vi "GUI_Lcave_AmplifierCams.vi"() -> ()   [LabVIEW 2013]
uses:
  shared programs/GUI_Template/GUI_master/tcp_new_data_event.ctl
  shared programs/GUI_Template/GUI_master/tcp new data cluster.ctl
  GUI_Stage_Cameras/Controls/Crosshair type def.ctl
  <userlib>/_OpenG.lib/array/array.llb/Filter 1D Array with Scalar (String)__ogtk.vi
panel:
  in  "Color Box":u32(colorbox)
  in  "TargetSize.Y::7":dbl=45.0 caption="y" min=2.0 max=3000.0 format="%#_6f"
  in  "TargetSize.X::7":dbl=47.0 caption="x" min=2.0 max=3000.0 format="%#_6f"
  in  "TargetSize.Y::6":dbl=45.0 caption="y" min=2.0 max=3000.0 format="%#_6f"
  in  "TargetSize.X::6":dbl=47.0 caption="x" min=2.0 max=3000.0 format="%#_6f"
  in  "TargetSize.Y::5":dbl=45.0 caption="y" min=2.0 max=3000.0 format="%#_6f"
  in  "TargetSize.X::5":dbl=47.0 caption="x" min=2.0 max=3000.0 format="%#_6f"
  in  "TargetSize.Y::4":dbl=45.0 caption="y" min=2.0 max=3000.0 format="%#_6f"
  in  "TargetSize.X::4":dbl=47.0 caption="x" min=2.0 max=3000.0 format="%#_6f"
  in  "TargetSize.Y::3":dbl=163.0 caption="y" min=2.0 max=3000.0 format="%#_6f"
  in  "TargetSize.X::3":dbl=152.0 caption="x" min=2.0 max=3000.0 format="%#_6f"
  in  "TargetSize.Y::2":dbl=74.0 caption="y" min=2.0 max=3000.0 format="%#_6f"
  in  "TargetSize.X::2":dbl=75.0 caption="x" min=2.0 max=3000.0 format="%#_6f"
  in  "active cams":string
  out "CCDs":string[](array[string])
  out "Cameras":T1
  in  "Target.Y::7":dbl=45.0 caption="y" min=0.0 max=2000.0 format="%#_6f"
  in  "Target.X::7":dbl=47.0 caption="x" min=0.0 max=2000.0 format="%#_6f"
  in  "Target.Y::6":dbl=45.0 caption="y" min=0.0 max=2000.0 format="%#_6f"
  in  "Target.X::6":dbl=47.0 caption="x" min=0.0 max=2000.0 format="%#_6f"
  in  "Target.Y::5":dbl=45.0 caption="y" min=0.0 max=2000.0 format="%#_6f"
  in  "Target.X::5":dbl=47.0 caption="x" min=0.0 max=2000.0 format="%#_6f"
  in  "Target.Y::4":dbl=45.0 caption="y" min=0.0 max=2000.0 format="%#_6f"
  in  "Target.X::4":dbl=47.0 caption="x" min=0.0 max=2000.0 format="%#_6f"
  in  "Target.Y::3":dbl=163.0 caption="y" min=0.0 max=2000.0 format="%#_6f"
  in  "Target.X::3":dbl=152.0 caption="x" min=0.0 max=2000.0 format="%#_6f"
  in  "Target.Y::2":dbl=74.0 caption="y" min=0.0 max=2000.0 format="%#_6f"
  in  "Target.X::2":dbl=75.0 caption="x" min=0.0 max=2000.0 format="%#_6f"
  out "error out":errorcluster
  out "image::7":T2(plugin-control) caption="GaiaImager2"
  in  "triggerdelay::7":dbl=0.001 caption="triggerdelay" min=0.0 max=0.09 format="%_4p"
  in  "triggerdelay::6":dbl=0.001 caption="triggerdelay" min=0.0 max=0.09 format="%_4p"
  in  "triggerdelay::5":dbl=0.001 caption="triggerdelay" min=0.0 max=0.09 format="%_4p"
  in  "triggerdelay::4":dbl=0.001 caption="triggerdelay" min=0.0 max=0.09 format="%_4p"
  in  "triggerdelay::3":dbl=0.001 caption="triggerdelay" min=0.0 max=0.09 format="%_4p"
  in  "triggerdelay::2":dbl=0.001 caption="triggerdelay" min=0.0 max=0.09 format="%_4p"
  in  "trigger::7":bool caption="Trigger"
  in  "centroidy::7":dbl=0.001 caption="centroid y" min=0.0 max=0.0 format="%_4f"
  in  "centroidx::7":dbl=0.001 caption="centroid x" min=0.0 max=0.0 format="%_4f"
  in  "exposure::7":dbl=0.001 caption="exposure" min=0.0001 max=1.0 format="%_4p"
  in  "GUIdevice 7":string="GaiaImager2"
  in  "trigger::6":bool caption="Trigger"
  in  "centroidy::6":dbl=0.001 caption="centroid y" min=0.0 max=0.0 format="%_4f"
  in  "centroidx::6":dbl=0.001 caption="centroid x" min=0.0 max=0.0 format="%_4f"
  in  "exposure::6":dbl=0.001 caption="exposure" min=0.0001 max=1.0 format="%_4p"
  out "image::6":T2(plugin-control) caption="BellaCam13_2"
  in  "GUIdevice 6":string="BellaCam13_2"
  in  "trigger::5":bool caption="Trigger"
  in  "centroidy::5":dbl=0.001 caption="centroid y" min=0.0 max=0.0 format="%_4f"
  in  "centroidx::5":dbl=0.001 caption="centroid x" min=0.0 max=0.0 format="%_4f"
  in  "exposure::5":dbl=0.001 caption="exposure" min=0.0001 max=1.0 format="%_4p"
  out "image::5":T2(plugin-control) caption="BellaCam16_3"
  in  "GUIdevice 5":string="BellaCam16_4"
  in  "trigger::4":bool caption="Trigger"
  in  "centroidy::4":dbl=0.001 caption="centroid y" min=0.0 max=0.0 format="%_4f"
  in  "centroidx::4":dbl=0.001 caption="centroid x" min=0.0 max=0.0 format="%_4f"
  in  "exposure::4":dbl=0.001 caption="exposure" min=0.0001 max=1.0 format="%_4p"
  out "image::4":T2(plugin-control) caption="BellaCam16_3"
  in  "GUIdevice 4":string="BellaCam16_3"
  in  "trigger::3":bool caption="Trigger"
  in  "centroidy::3":dbl=0.001 caption="centroid y" min=0.0 max=0.0 format="%_4f"
  in  "centroidx::3":dbl=0.001 caption="centroid x" min=0.0 max=0.0 format="%_4f"
  in  "exposure::3":dbl=0.001 caption="exposure" min=0.0001 max=1.0 format="%_4p"
  out "image::3":T2(plugin-control) caption="BellaCam16_2"
  in  "GUIdevice 3":string="BellaCam16_2"
  in  "trigger::2":bool caption="Trigger"
  in  "centroidy::2":dbl=0.001 caption="centroid y" min=0.0 max=0.0 format="%_4f"
  in  "centroidx::2":dbl=0.001 caption="centroid x" min=0.0 max=0.0 format="%_4f"
  in  "exposure::2":dbl=0.001 caption="exposure" min=0.0001 max=1.0 format="%_4p"
  out "image::2":T2(plugin-control) caption="BellaCam16_1"
  in  "GUIdevice 2":string="BellaCam16_1"
  out "tcp data event":T3
  in  "Refresh Button":bool caption="Update Crosshairs"
  in  "Select device":string(combo)="FrogHPD"
  in  "stop":bool
  in  "GUIdevice 1":string="HPD_CCD"
  # "XHair location"
  # "XHair size"
  # "XHair location"
  # "XHair size"
  # "XHair location"
  # "XHair size"
  # "XHair location"
  # "XHair size"
  # "XHair location"
  # "XHair size"
  # "XHair location"
  # "XHair size"
  # "XHair location"
  # "XHair size"
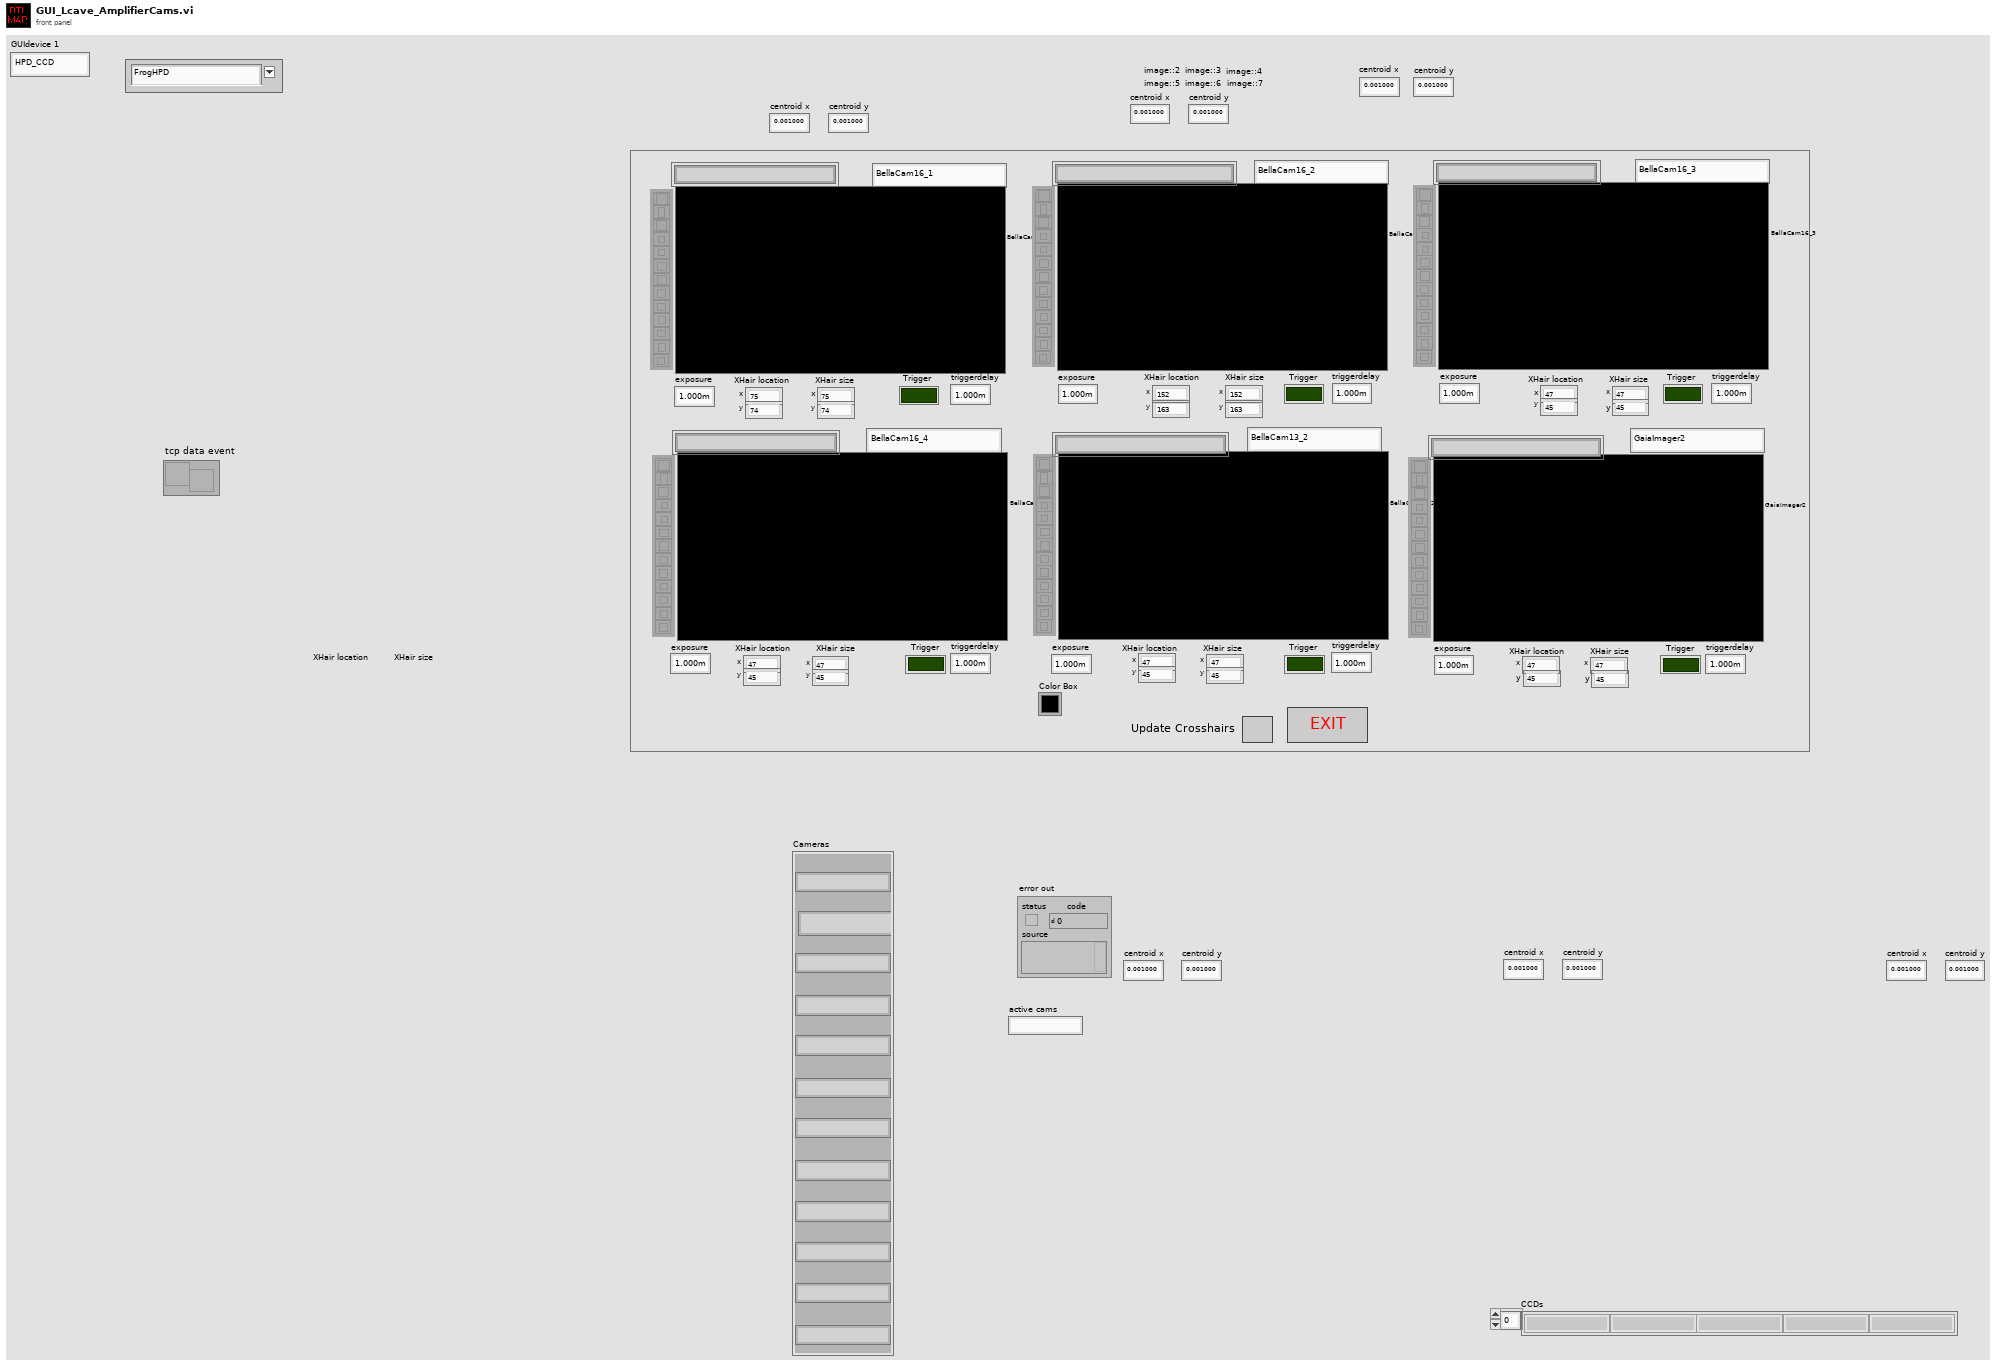
[diagram p1: front panel]
types:
  T1 = cluster{"[0]":string, "[1]":string, "[2]":string, "[3]":string, "[4]":string, "[5]":string, "[6]":string, "[7]":string, "[8]":string, "[8] 2":string, "[8] 3":string, "[8] 4":string}
  T2 = typedef "IMAQ Image.ctl" = refnum<image>
  T3 = typedef "tcp_new_data_event.ctl" = refnum<user-event>
  T4 = typedef "Image Type" = u32
  T5 = cluster{"TargetSize.X::2":refnum<vi>, "TargetSize.Y::2":refnum<vi>}
  T6 = cluster{"TargetSize.X::3":refnum<vi>, "TargetSize.Y::3":refnum<vi>}
  T7 = cluster{"TargetSize.X::4":refnum<vi>, "TargetSize.Y::4":refnum<vi>}
  T8 = cluster{"TargetSize.X::5":refnum<vi>, "TargetSize.Y::5":refnum<vi>}
  T9 = cluster{"TargetSize.X::6":refnum<vi>, "TargetSize.Y::6":refnum<vi>}
  T10 = cluster{"TargetSize.X::7":refnum<vi>, "TargetSize.Y::7":refnum<vi>}
  T11 = cluster{"Target.X::2":refnum<vi>, "Target.Y::2":refnum<vi>}
  T12 = cluster{"Target.X::3":refnum<vi>, "Target.Y::3":refnum<vi>}
  T13 = cluster{"Target.X::4":refnum<vi>, "Target.Y::4":refnum<vi>}
  T14 = cluster{"Target.X::5":refnum<vi>, "Target.Y::5":refnum<vi>}
  T15 = cluster{"Target.X::6":refnum<vi>, "Target.Y::6":refnum<vi>}
  T16 = cluster{"Target.X::7":refnum<vi>, "Target.Y::7":refnum<vi>}
  T17 = cluster{"[0]":string, "[1]":string, "[2]":string, "[3]":string, "[4]":string, "[5]":string, "[6]":string, "[7]":string, "[8]":string, "[9]":string, "[10]":string, "[11]":string}
  T18 = cluster{"TargetSize.X::7":refnum<vi>, "TargetSize.Y::7":refnum<vi>}[]
  T19 = cluster{"Target.X::7":refnum<vi>, "Target.Y::7":refnum<vi>}[]
  T20 = typedef "Crosshair type def.ctl" = cluster{"Draw":bool, "Target":cluster{"x":dbl, "y":dbl}, "Size":cluster{"x":dbl, "y":dbl}, "Angle":dbl, "Color":u32}
  T21 = cluster{"Left":i32, "Top":i32, "Right":i32, "Bottom":i32}
  T22 = enum32{"invalid app kind", "Development System", "Run Time System", "Student Edition", "Embedded LabVIEW", "Evaluation", "Custom"}
  T23 = typedef "tcp new data cluster.ctl" = cluster{"EventEnum":enum16{"new data", "connection status update"}, "Device name":string}
  T24 = enum32{"Invalid", "Standard", "Closed", "Hidden", "Minimized", "Maximized"}
  T25 = cluster{"Core":cluster{"Current VI Reference":refnum<vi>, "Close Panel on Exit?":bool}, "Your Boolean data":bool, "active cams":string, "SuperGUI":cluster{"STOP queue":refnum<queue>, "SuperGUI ref":refnum<vi>}}
  T26 = cluster{"STOP queue":refnum<queue>, "SuperGUI ref":refnum<vi>}
  T27 = cluster{"Current VI Reference":refnum<vi>, "Close Panel on Exit?":bool}
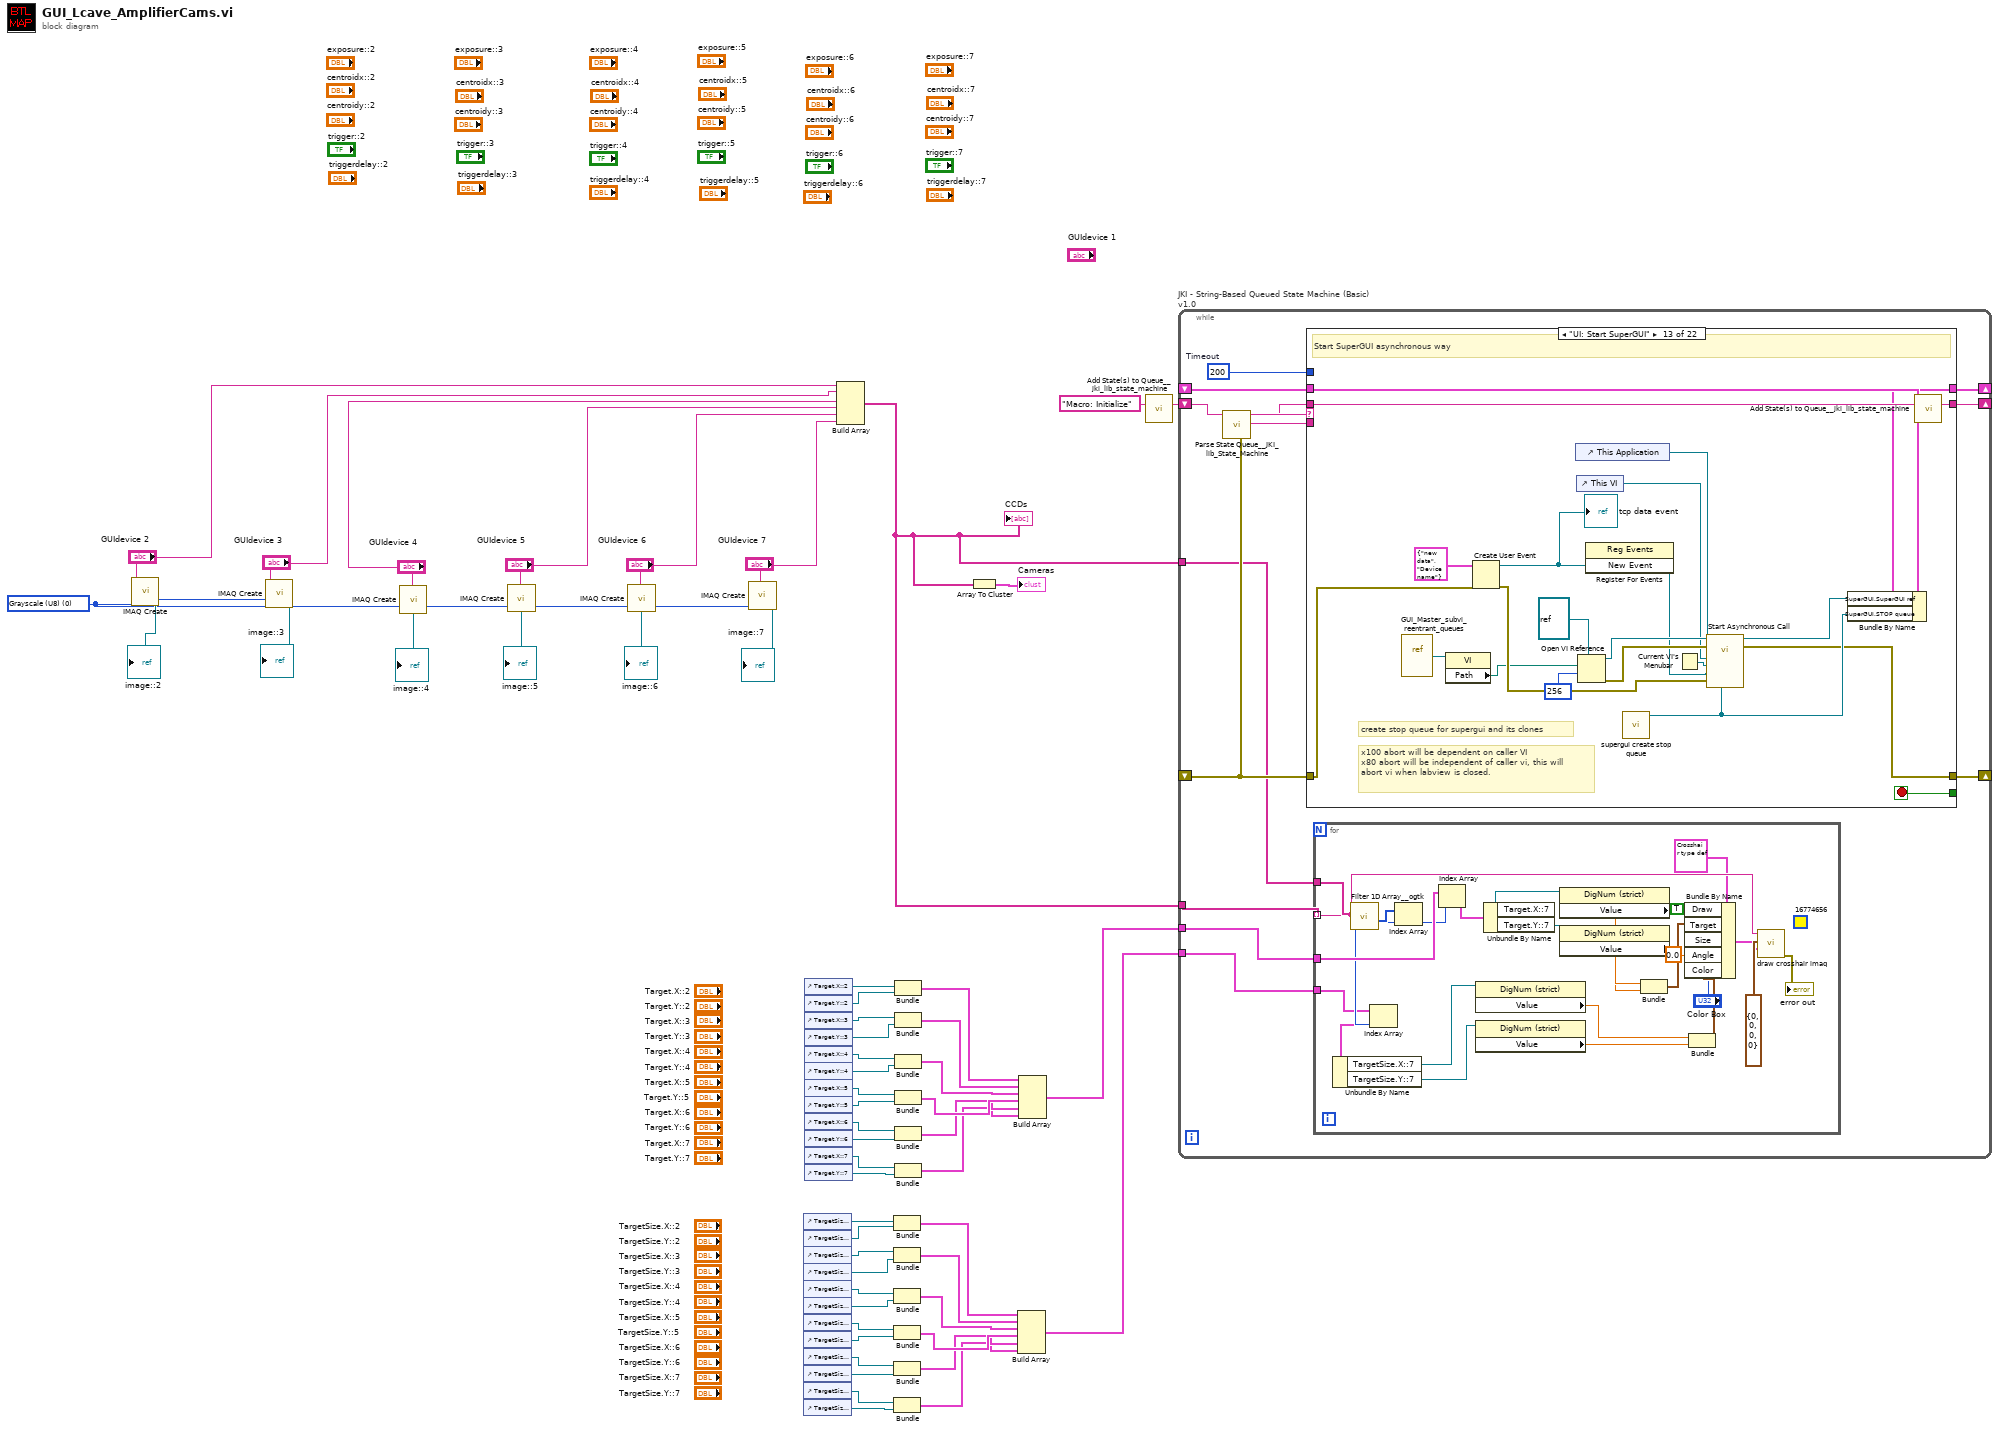
[diagram p0: block diagram]
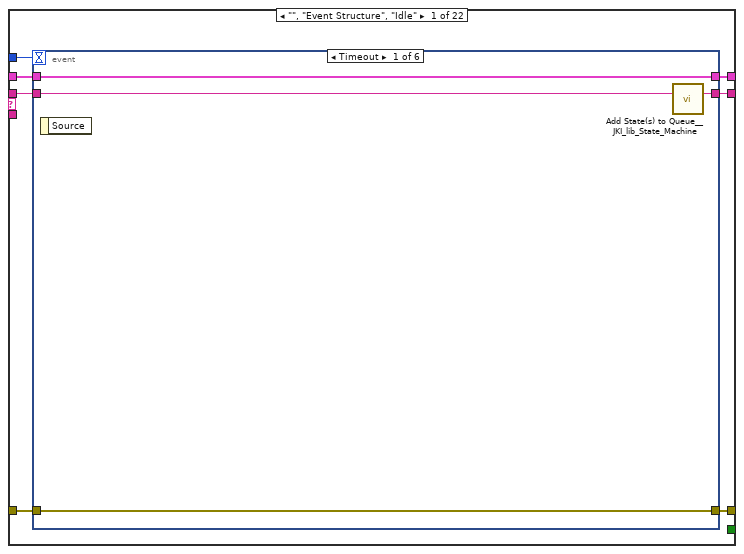
[diagram p2: hidden frame]
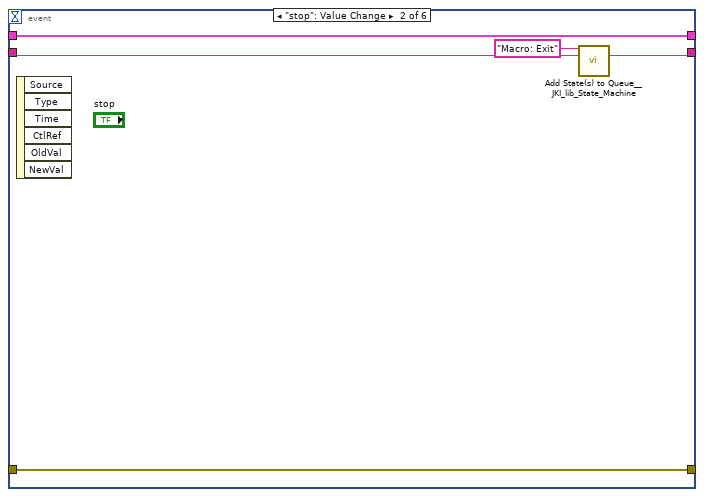
[diagram p3: hidden frame]
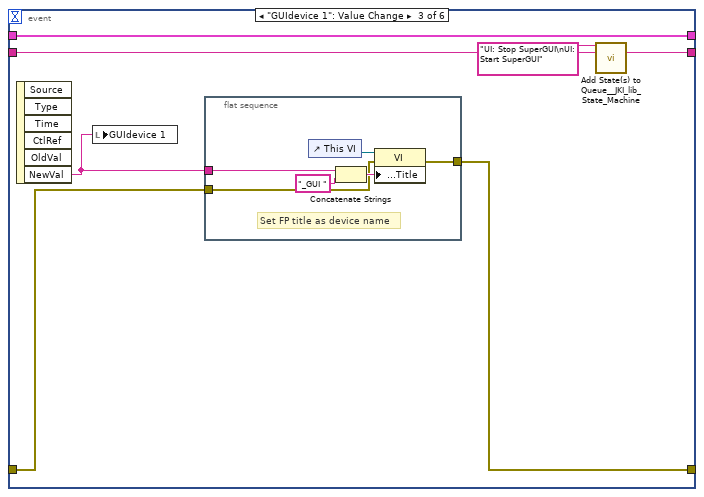
[diagram p4: hidden frame]
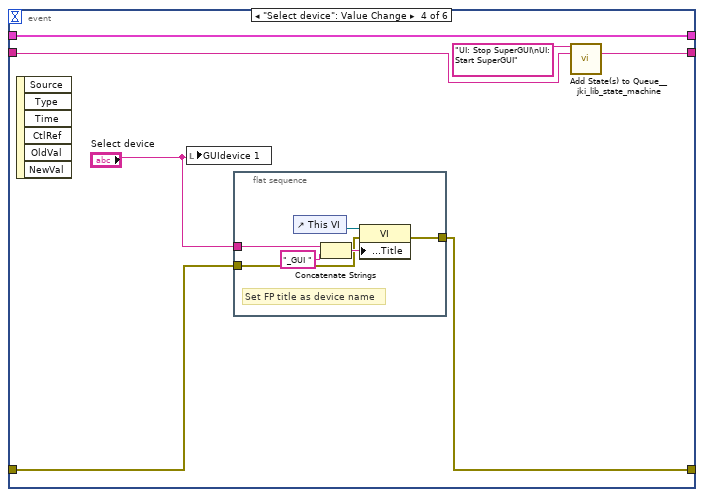
[diagram p5: hidden frame]
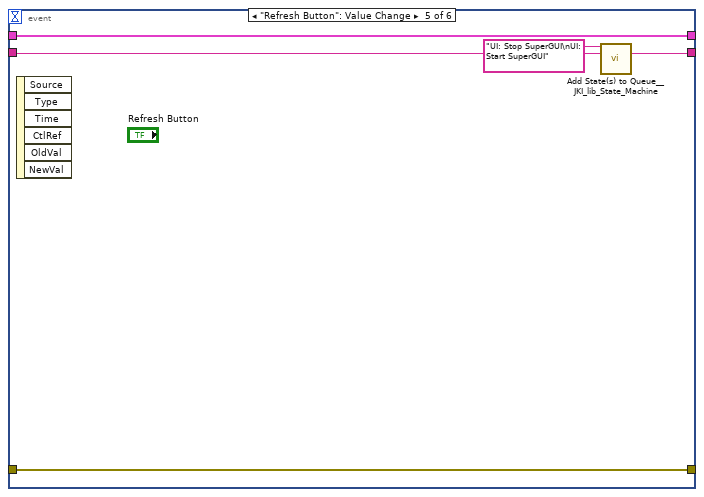
[diagram p6: hidden frame]
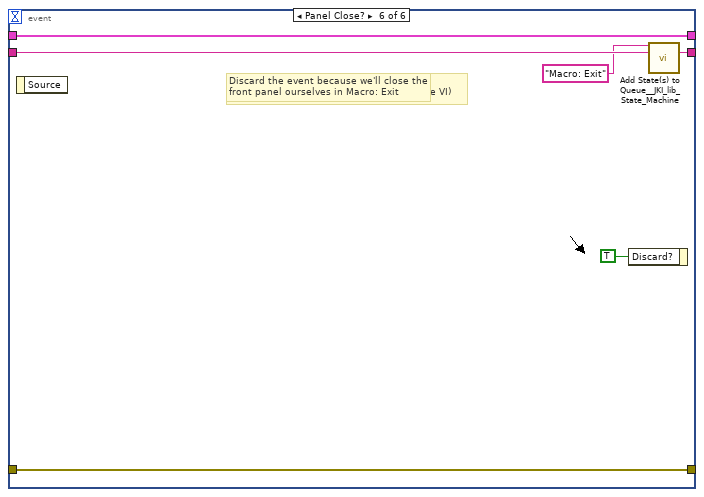
[diagram p7: hidden frame]
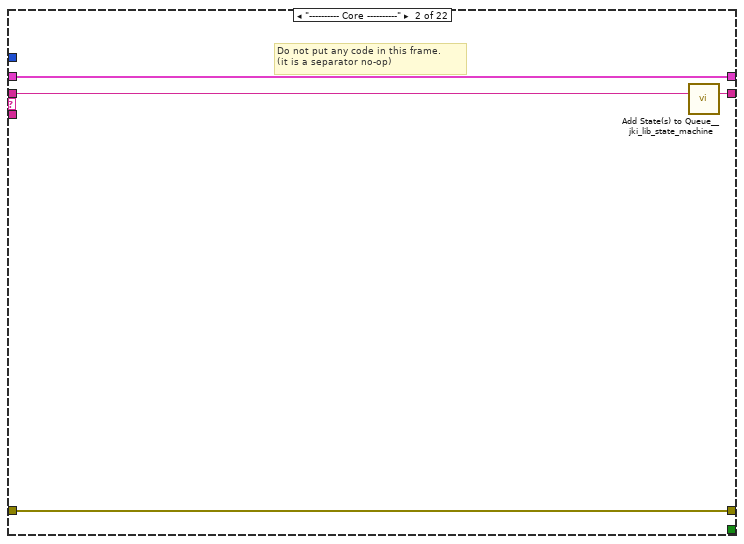
[diagram p8: hidden frame]
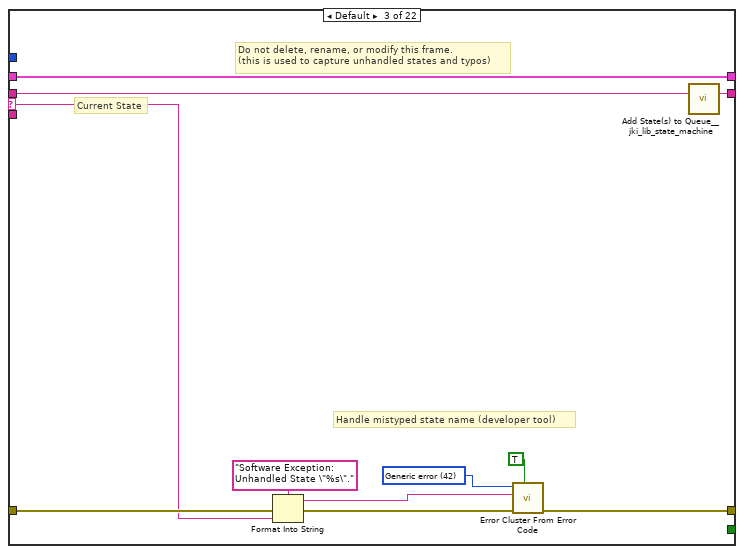
[diagram p9: hidden frame]
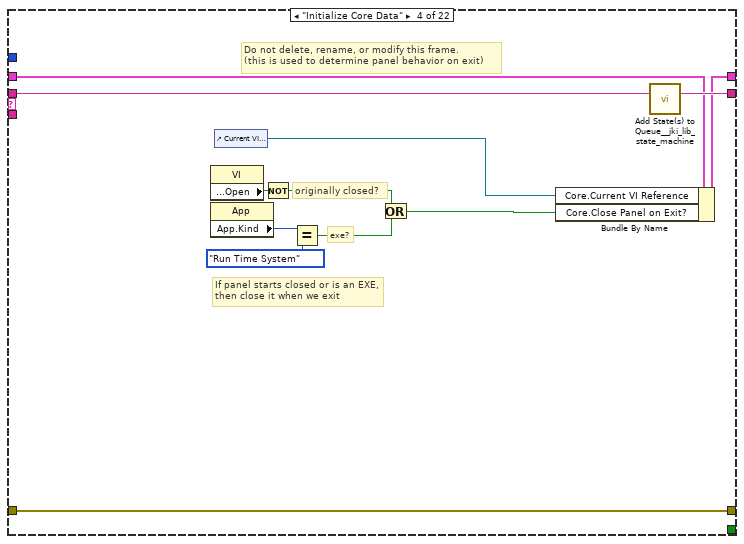
[diagram p10: hidden frame]
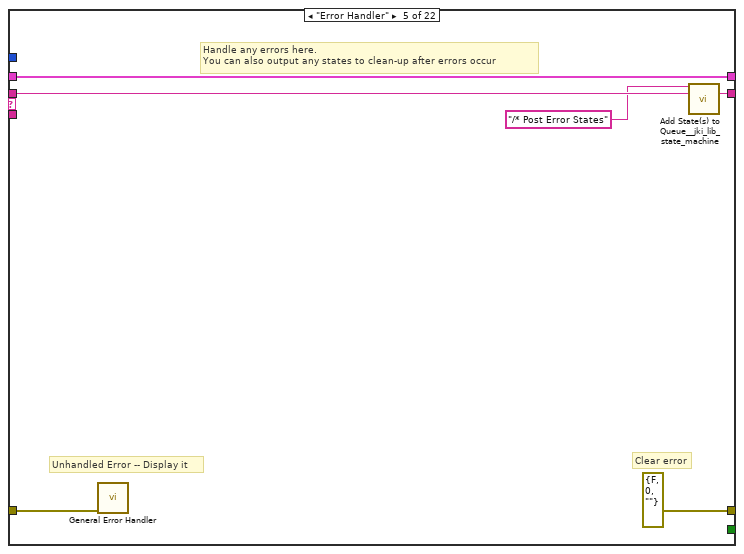
[diagram p11: hidden frame]
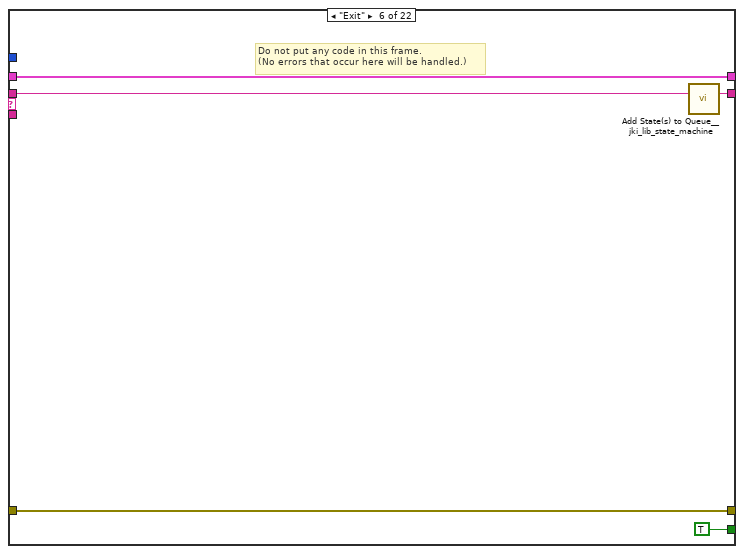
[diagram p12: hidden frame]
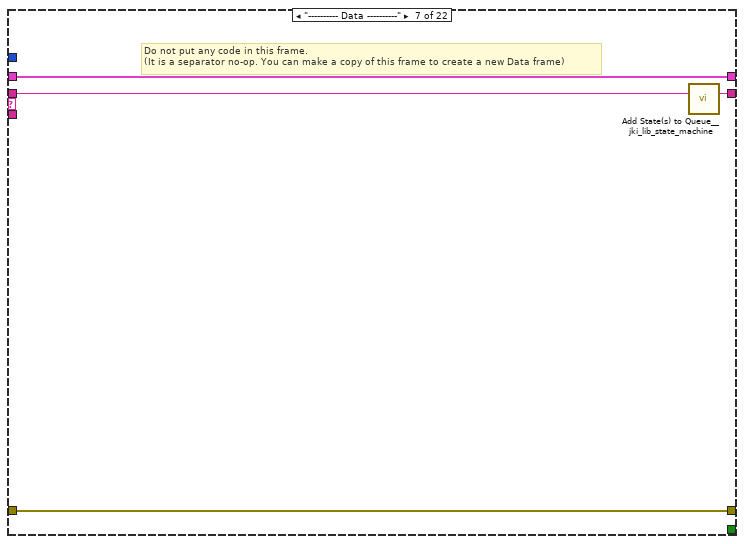
[diagram p13: hidden frame]
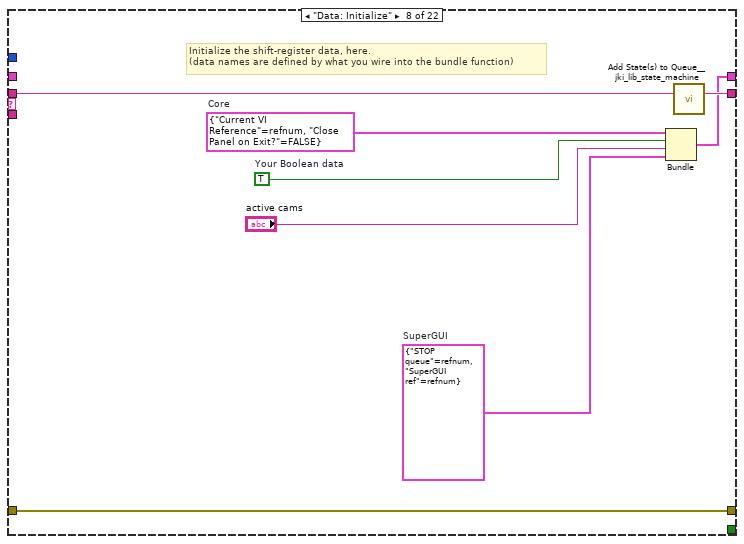
[diagram p14: hidden frame]
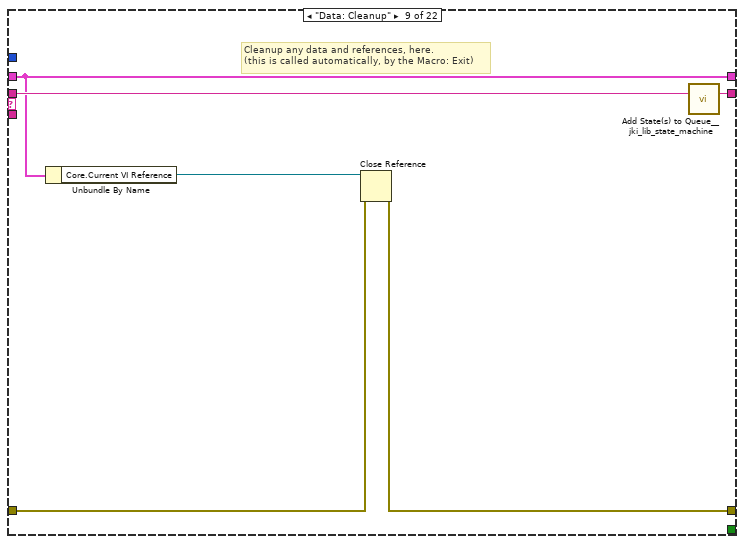
[diagram p15: hidden frame]
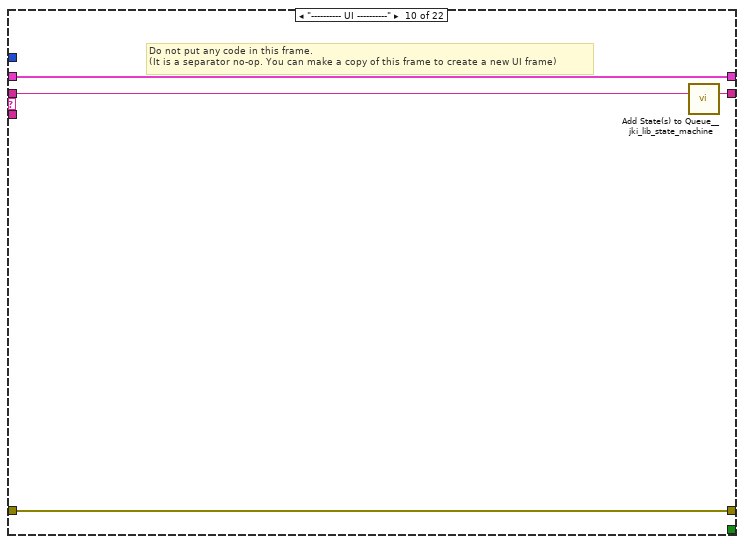
[diagram p16: hidden frame]
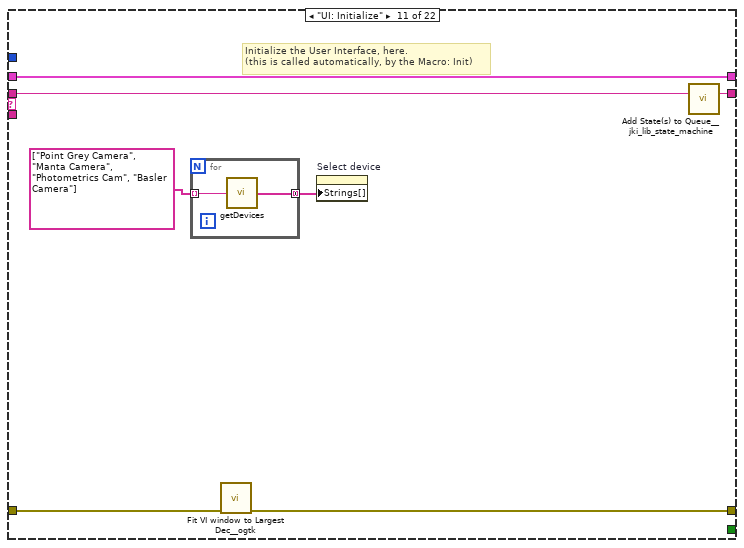
[diagram p17: hidden frame]
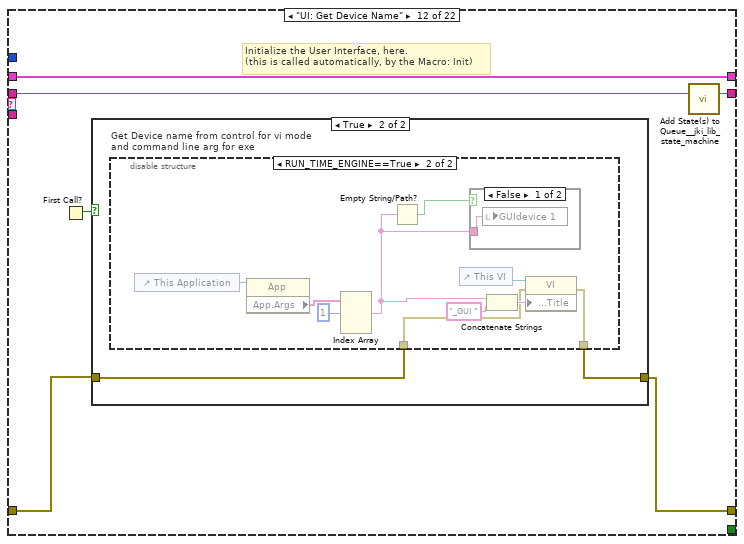
[diagram p18: hidden frame]
diagram:
  w48 = T4 0 items=["Grayscale (U8)", "Grayscale (I16)", "Grayscale (SGL)", "Complex (CSG)", "RGB (U32)", "HSL (U32)", "RGB (U64)", "Grayscale (U16)"] ("Image Type")
  n1 = call "IMAQ Create"("Image Name"="GUIdevice 2", "Image Type"=w48) -> ("New Image"=→"image::2":T2)  [unwired: 3 in, 1 out]
  n2 = call "IMAQ Create"("Image Name"="GUIdevice 3", "Image Type"=w48) -> ("New Image"=→"image::3":T2)  [unwired: 3 in, 1 out]
  n3 = call "IMAQ Create"("Image Name"="GUIdevice 4", "Image Type"=w48) -> ("New Image"=→"image::4":T2)  [unwired: 3 in, 1 out]
  n4 = call "IMAQ Create"("Image Name"="GUIdevice 5", "Image Type"=w48) -> ("New Image"=→"image::5":T2)  [unwired: 3 in, 1 out]
  n5 = call "IMAQ Create"("Image Name"="GUIdevice 6", "Image Type"=w48) -> ("New Image"=→"image::6":T2)  [unwired: 3 in, 1 out]
  n6 = call "IMAQ Create"("Image Name"="GUIdevice 7", "Image Type"=w48) -> ("New Image"=→"image::7":T2)  [unwired: 3 in, 1 out]
  n7 = control-ref of="TargetSize.X::2"() -> (w19:refnum<vi>)
  n8 = control-ref of="TargetSize.Y::2"() -> (w18:refnum<vi>)
  n9 = control-ref of="TargetSize.X::3"() -> (w17:refnum<vi>)
  n10 = control-ref of="TargetSize.Y::3"() -> (w16:refnum<vi>)
  n11 = control-ref of="TargetSize.X::4"() -> (w15:refnum<vi>)
  n12 = control-ref of="TargetSize.Y::4"() -> (w14:refnum<vi>)
  n13 = control-ref of="TargetSize.X::5"() -> (w13:refnum<vi>)
  n14 = control-ref of="TargetSize.Y::5"() -> (w12:refnum<vi>)
  n15 = control-ref of="TargetSize.X::6"() -> (w11:refnum<vi>)
  n16 = control-ref of="TargetSize.Y::6"() -> (w10:refnum<vi>)
  n17 = control-ref of="TargetSize.X::7"() -> (w9:refnum<vi>)
  n18 = control-ref of="TargetSize.Y::7"() -> (w8:refnum<vi>)
  n19 = control-ref of="Target.X::2"() -> (w46:refnum<vi>)
  n20 = control-ref of="Target.Y::2"() -> (w45:refnum<vi>)
  n21 = control-ref of="Target.X::3"() -> (w44:refnum<vi>)
  n22 = control-ref of="Target.Y::3"() -> (w43:refnum<vi>)
  n23 = control-ref of="Target.X::4"() -> (w42:refnum<vi>)
  n24 = control-ref of="Target.Y::4"() -> (w41:refnum<vi>)
  n25 = control-ref of="Target.X::5"() -> (w40:refnum<vi>)
  n26 = control-ref of="Target.Y::5"() -> (w39:refnum<vi>)
  n27 = control-ref of="Target.X::6"() -> (w38:refnum<vi>)
  n28 = control-ref of="Target.Y::6"() -> (w37:refnum<vi>)
  n29 = control-ref of="Target.X::7"() -> (w36:refnum<vi>)
  n30 = control-ref of="Target.Y::7"() -> (w35:refnum<vi>)
  n31 = Build Array("GUIdevice 2", "GUIdevice 3", "GUIdevice 4", "GUIdevice 5", "GUIdevice 6", "GUIdevice 7") -> (w20:string[])
  "CCDs" <- w20
  n32 = Bundle("TargetSize.X::2"=w19, "TargetSize.Y::2"=w18) -> (w7:T5)  [unwired: 1 in]
  n33 = Bundle("TargetSize.X::3"=w17, "TargetSize.Y::3"=w16) -> (w6:T6)  [unwired: 1 in]
  n34 = Bundle("TargetSize.X::4"=w15, "TargetSize.Y::4"=w14) -> (w2:T7)  [unwired: 1 in]
  n35 = Bundle("TargetSize.X::5"=w13, "TargetSize.Y::5"=w12) -> (w5:T8)  [unwired: 1 in]
  n36 = Bundle("TargetSize.X::6"=w11, "TargetSize.Y::6"=w10) -> (w4:T9)  [unwired: 1 in]
  n37 = Bundle("TargetSize.X::7"=w9, "TargetSize.Y::7"=w8) -> (w3:T10)  [unwired: 1 in]
  n38 = Bundle("Target.X::2"=w46, "Target.Y::2"=w45) -> (w34:T11)  [unwired: 1 in]
  n39 = Bundle("Target.X::3"=w44, "Target.Y::3"=w43) -> (w33:T12)  [unwired: 1 in]
  n40 = Bundle("Target.X::4"=w42, "Target.Y::4"=w41) -> (w29:T13)  [unwired: 1 in]
  n41 = Bundle("Target.X::5"=w40, "Target.Y::5"=w39) -> (w32:T14)  [unwired: 1 in]
  n42 = Bundle("Target.X::6"=w38, "Target.Y::6"=w37) -> (w31:T15)  [unwired: 1 in]
  n43 = Bundle("Target.X::7"=w36, "Target.Y::7"=w35) -> (w30:T16)  [unwired: 1 in]
  n44 = Array To Cluster(array=w20) -> (cluster=→"Cameras":T17)
  n45 = Build Array(w7, w6, w2, w5, w4, w3) -> (w1:T18)
  n46 = Build Array(w34, w33, w29, w32, w31, w30) -> (w28:T19)
  n47 = call <vilib>:"Add State(s) to Queue__jki_lib_state_machine.vi"("State(s) in (\"\")"="Macro: Initialize") -> ("States Out"=w55:string)  [unwired: 14 in]
  n48 = while "JKI - String-Based Queued State Machine (Basic) v1.0" {
    shift-right: [w63] -> _
    shift-left: _ -> [w58]
    shift-right: [w66] -> _
    shift-left: _ -> [w61]
    shift-right: [w65] -> _
    shift-left: w55 -> [w67]
    tunnel: w28 -> [w60]
    tunnel: w20 -> [w59]
    tunnel: w20 -> [w57]
    tunnel: w1 -> [w56]
    stop <- w64 stop-if-true
    w62 = 200  # Timeout
    n49 = call <vilib>:"Parse State Queue__JKI_lib_State_Machine.vi"("State Queue"=w67, "Error In (no error)"=w61) -> ("Remaining States"=w69:string, "Current State"=w70:string, "Arguments"=w68:string)  [unwired: 11 in]
    n50 = case shown="\"UI: Start SuperGUI\"" w70 {
      selector: w70 -> [_ _ w153 _ _ _ _ _ _ _ _ _ _ _ _ _ _ _ _ _ _ _]
      tunnel: w69 -> [w102 w152 w157 w175 w181 w186 w190 w198 w204 w208 w215 w223 w258 w266 w272 w283 w309 w314 w324 w328 w332 w336]
      tunnel: w68 -> [_ _ _ _ _ _ _ _ _ _ _ _ _ _ w267 w277 _ _ _ _ _ _]
      tunnel: w58 -> [w100 w149 w155 w166 w178 w184 w187 _ w199 w205 w213 w221 w249 w261 w270 w279 w306 w311 w321 w325 w329 w333]
      tunnel: [w99 w150 w159 w172 errorcluster {"status"=FALSE, "code"=0, "source"=""} ("error out") w183 w188 w195 w200 w206 w211 w218 w242 w259 w268 w280 w307 w312 w322 w326 w330 w334] -> w66
      tunnel: w61 -> [w98 w150 w158 w172 w177 w183 w188 w195 w201 w206 w212 w219 w243 w260 w269 w281 w307 w312 w322 w326 w330 w334]
      tunnel: [w101 w151 w156 w174 w180 w185 w189 w197 w203 w207 w214 w222 w257 w265 w271 w282 w308 w313 w323 w327 w331 w335] -> w65
      tunnel: [_ _ _ _ _ TRUE _ _ _ _ _ _ _ _ _ _ _ _ _ _ _ _] -> w64
      tunnel: [w97 w149 w155 w173 w178 w184 w187 w196 w199 w205 w213 w221 w248 w261 w270 w279 w306 w311 w321 w325 w329 w333] -> w63
      tunnel: w62 -> [w96 _ _ _ _ _ _ _ _ _ _ _ _ _ _ _ _ _ _ _ _ _]
      frame "", "Event Structure", "Idle" {
        n51 = event shown="[0] Timeout" {
          selector: _ -> [_ _ _ _ _ _]
          dyn-events: _ -> [_ _ _ _ _ _]
          timeout: w96 -> [_ _ _ _ _ _]
          tunnel: w102 -> [w106 w109 w115 w127 w140 w148]
          tunnel: [w105 w108 w114 w126 w139 w147] -> w101
          tunnel: w100 -> [w103 w111 w118 w131 w142 w145]
          tunnel: [w104 w110 w116 w129 w141 w146] -> w99
          tunnel: w98 -> [w104 w110 w117 w130 w141 w146]
          tunnel: [w103 w111 w118 w131 w142 w145] -> w97
          event Timeout {
            n52 = event-data() -> ()  [unwired: 1 in, 1 out]
            n53 = call <vilib>:"Add State(s) to Queue__JKI_lib_State_Machine.vi"("State(s) in (\"\")"=w106) -> ("States Out"=w105:string)  [unwired: 14 in]
          }
          event "stop": Value Change {
            n54 = event-data() -> ()  [unwired: 1 in, 6 out]
            n55 = call <vilib>:"Add State(s) to Queue__JKI_lib_State_Machine.vi"("State(s) in Front (\"\")"="Macro: Exit", "State(s) in (\"\")"=w109) -> ("States Out"=w108:string)  [unwired: 13 in]
          }
          event "GUIdevice 1": Value Change {
            n56 = event-data() -> ("NewVal"=w112:string)  [unwired: 1 in, 5 out]
            n57 = local write "GUIdevice 1"(w112) -> ()
            n58 = flat-sequence {
              tunnel: [w121] -> w116
              tunnel: w117 -> [w120]
              tunnel: w112 -> [w119]
              frame #0 {
                # "Set FP title as device name"
                n59 = control-ref of="This VI"() -> (w124:refnum<vi>)
                n60 = Concatenate Strings(w119, "_GUI ") -> (w123:string)
                n61 = property class="VI"(reference=w124, error in=w120, "Front Panel.Title"=w123) -> (error out=w121:errorcluster)  [unwired: 1 out]
              }
            }
            n62 = call <vilib>:"Add State(s) to Queue__JKI_lib_State_Machine.vi"("State(s) in Front (\"\")"="UI: Stop SuperGUI\nUI: Start SuperGUI", "State(s) in (\"\")"=w115) -> ("States Out"=w114:string)  [unwired: 13 in]
          }
          event "Select device": Value Change {
            n63 = event-data() -> ()  [unwired: 1 in, 6 out]
            n64 = local write "GUIdevice 1"("Select device") -> ()
            n65 = flat-sequence {
              tunnel: [w134] -> w129
              tunnel: w130 -> [w133]
              tunnel: "Select device" -> [w132]
              frame #0 {
                # "Set FP title as device name"
                n66 = control-ref of="This VI"() -> (w137:refnum<vi>)
                n67 = Concatenate Strings(w132, "_GUI ") -> (w136:string)
                n68 = property class="VI"(reference=w137, error in=w133, "Front Panel.Title"=w136) -> (error out=w134:errorcluster)  [unwired: 1 out]
              }
            }
            n69 = call <vilib>:"Add State(s) to Queue__jki_lib_state_machine.vi"("State(s) in Front (\"\")"="UI: Stop SuperGUI\nUI: Start SuperGUI", "State(s) in (\"\")"=w127) -> ("States Out"=w126:string)  [unwired: 13 in]
          }
          event "Refresh Button": Value Change {
            n70 = event-data() -> ()  [unwired: 1 in, 6 out]
            n71 = call <vilib>:"Add State(s) to Queue__JKI_lib_State_Machine.vi"("State(s) in Front (\"\")"="UI: Stop SuperGUI\nUI: Start SuperGUI", "State(s) in (\"\")"=w140) -> ("States Out"=w139:string)  [unwired: 13 in]
          }
          event Panel Close? {
            # "Discard the event because we'll close the front panel ourselves in Macro: Exit"
            # "Close Panel button (pressed) Event\n(this executes Macro: Exit to terminate the VI)"
            n72 = event-data() -> ()  [unwired: 1 in, 1 out]
            n73 = event-data("Discard?"=TRUE) -> ()  [unwired: 1 in, 1 out]
            n74 = call <vilib>:"Add State(s) to Queue__JKI_lib_State_Machine.vi"("State(s) in Front (\"\")"="Macro: Exit", "State(s) in (\"\")"=w148) -> ("States Out"=w147:string)  [unwired: 13 in]
          }
        }
      }
      frame "---------- Core ----------" {
        # "Do not put any code in this frame.\n(it is a separator no-op)"
        n75 = call <vilib>:"Add State(s) to Queue__jki_lib_state_machine.vi"("State(s) in (\"\")"=w152) -> ("States Out"=w151:string)  [unwired: 14 in]
      }
      frame Default {
        w162 = 42 items=["No error", "Argument error", "Memory is full", "Out of zone", "End of file", "File already open", "Generic file I/O error", "File not found", "File permission error", "Disk is full", "Duplicate path", "Too many files open", "System feature not enabled", "Resource file not found", "Cannot add resource", "Resource not found", "Image not found", "Image memory error", "Pen does not exist", "Config type invalid", "Config token not found", "Config parse error", "Config memory error", "Bad external code format", "Bad external code offset", "External code not present", "Null window", "Destroy window error", "Null menu", "Print aborted", "Bad print record", "Print driver error", "Windows error during printing", "Memory error during printing", "Print dialog error", "Generic print error", "Invalid device refnum", "Device not found", "Device parameter error", "Device unit error", "Cannot open device", "Device call aborted", "Generic error", "Cancelled by user", "Object ID too low", "Object ID too high", "Object not in heap", "Unknown heap", "Unknown object (invalid DefProc)", "Unknown object (DefProc not in table)", "Message out of range", "Invalid (null) method", "Unknown message", "Manager call not supported", "Bad address", "Network operation in progress", "Network operation timed out", "Connection is busy", "Network attribute not supported", "Network error", "Address in use", "System out of memory", "Connection aborted", "Connection refused", "Not connected", "Already connected", "Connection closed", "Initialization error (interapplication manager)", "Bad occurrence", "Wait on unbound occurrence handler", "Occurrence queue overflow", "Datalog type conflict", "Unused", "Unrecognized type (interapplication manager)", "Memory corrupt", "Failed to make temporary DLL", "Old CIN version", "Drag socket not found", "Failed to load drop-object", "Failed to register OLE object", "Failed to release OLE object", "Format specifier type mismatch", "Unknown format specifier", "Too few format specifiers", "Too many format specifiers", "Scan failed", "Newer CIN version", "Error converting to variant", "Runtime menu error", "Password tampered", "Variant attribute not found", "Incompatible variant data type", "Event data is not available", "Event Store is not present", "Occurrence is not found", "Event Queue is not created", "Event info is not available", "Refnum passed is NULL", "Error retrieving Class GUID", "Error retrieving CoClass GUID", "Error retrieving TypeLib GUID.", "Bad built application magic bytes.", "Specific driver is different from the specific driver associated with the Logical Name.", "There is no session opened to the class driver.", "Max Error", "MAX - Error with config objects", "MAX - Error loading configuration", "MAX - Group not supported"]
        # "Current State"
        # "Do not delete, rename, or modify this frame.\n(this is used to capture unhandled states and typos)"
        # "Handle mistyped state name (developer tool)"
        n76 = Format Into String(format string="Software Exception: Unhandled State \"%s\"." ("message"), error in=w158, w153) -> (resulting string=w161:string, error out=w160:errorcluster)  [unwired: 1 in]
        n77 = call <vilib>:"Error Cluster From Error Code.vi"("show call chain? (False)"=TRUE, "error in (no error)"=w160, "error message (\"\")"=w161, "error code (0)"=w162) -> ("error out"=w159:errorcluster)  [unwired: 5 in]
        n78 = call <vilib>:"Add State(s) to Queue__jki_lib_state_machine.vi"("State(s) in (\"\")"=w157) -> ("States Out"=w156:string)  [unwired: 14 in]
      }
      frame "Initialize Core Data" {
        # "Do not delete, rename, or modify this frame.\n(this is used to determine panel behavior on exit)"
        # "originally closed?"
        # "exe?"
        # "If panel starts closed or is an EXE, then close it when we exit"
        n79 = property class="VI"() -> ("Front Panel.Open"=w171:bool)  [unwired: 2 in, 2 out]
        n80 = property class="App"() -> ("App.Kind"=w170:T22)  [unwired: 2 in, 2 out]
        n81 = control-ref of="Current VI Reference"() -> (w164:refnum<vi>)
        n82 = Not(x=w171) -> (.not. x?=w168:bool)
        n83 = Equal?(x=w170, y=T22."Run Time System" ("Application:Kind")) -> (x = y?=w167:bool)
        n84 = Or(x=w168, y=w167) -> (x .or. y?=w165:bool)
        n85 = Bundle By Name(cluster=w166, "Core.Current VI Reference"=w164, "Core.Close Panel on Exit?"=w165) -> (w173:T25)
        n86 = call <vilib>:"Add State(s) to Queue__jki_lib_state_machine.vi"("State(s) in (\"\")"=w175) -> ("States Out"=w174:string)  [unwired: 14 in]
      }
      frame "Error Handler" {
        # "Unhandled Error -- Display it"
        # "Handle any errors here.\nYou can also output any states to clean-up after errors occur"
        # "Clear error"
        n87 = call <vilib>:"General Error Handler.vi"("error in (no error)"=w177) -> ()  [unwired: 10 in, 5 out]
        n88 = call <vilib>:"Add State(s) to Queue__jki_lib_state_machine.vi"("State(s) in Front (\"\")"="/* Post Error States", "State(s) in (\"\")"=w181) -> ("States Out"=w180:string)  [unwired: 13 in]
      }
      frame "Exit" {
        # "Do not put any code in this frame.\n(No errors that occur here will be handled.)"
        n89 = call <vilib>:"Add State(s) to Queue__jki_lib_state_machine.vi"("State(s) in (\"\")"=w186) -> ("States Out"=w185:string)  [unwired: 14 in]
      }
      frame "---------- Data ----------" {
        # "Do not put any code in this frame.\n(It is a separator no-op. You can make a copy of this frame to create a new Data frame)"
        n90 = call <vilib>:"Add State(s) to Queue__jki_lib_state_machine.vi"("State(s) in (\"\")"=w190) -> ("States Out"=w189:string)  [unwired: 14 in]
      }
      frame "Data: Initialize" {
        w191 = T26 {"STOP queue"=refnum, "SuperGUI ref"=refnum}  # SuperGUI
        w192 = T27 {"Current VI Reference"=refnum, "Close Panel on Exit?"=FALSE}  # Core
        w194 = TRUE  # Your Boolean data
        # "Initialize the shift-register data, here.\n(data names are defined by what you wire into the bundle function)"
        n91 = Bundle("Core"=w192, "Your Boolean data"=w194, "active cams"="active cams", "SuperGUI"=w191) -> (w196:T25)  [unwired: 1 in]
        n92 = call <vilib>:"Add State(s) to Queue__jki_lib_state_machine.vi"("State(s) in (\"\")"=w198) -> ("States Out"=w197:string)  [unwired: 14 in]
      }
      frame "Data: Cleanup" {
        # "Cleanup any data and references, here.\n(this is called automatically, by the Macro: Exit)"
        n93 = Unbundle By Name(w199) -> ("Core.Current VI Reference"=w202:refnum<vi>)
        n94 = Close Reference(reference=w202, error in (no error)=w201) -> (error out=w200:errorcluster)
        n95 = call <vilib>:"Add State(s) to Queue__jki_lib_state_machine.vi"("State(s) in (\"\")"=w204) -> ("States Out"=w203:string)  [unwired: 14 in]
      }
      frame "---------- UI ----------" {
        # "Do not put any code in this frame.\n(It is a separator no-op. You can make a copy of this frame to create a new UI frame)"
        n96 = call <vilib>:"Add State(s) to Queue__jki_lib_state_machine.vi"("State(s) in (\"\")"=w208) -> ("States Out"=w207:string)  [unwired: 14 in]
      }
      frame "UI: Initialize" {
        # "Initialize the User Interface, here.\n(this is called automatically, by the Macro: Init)"
        n97 = for {
          tunnel: string[] ["Point Grey Camera", "Manta Camera", "Photometrics Cam", "Basler Camera"] -> [w217] mode=indexing
          tunnel: [w216] -> w209 mode=concatenating
          n98 = call "getDevices.vi"("Device Class"=w217) -> ("All Devices"=w216:string[])
        }
        n99 = call <userlib>:"Fit VI window to Largest Dec__ogtk.vi"("error in (no error)"=w212) -> ("error out"=w211:errorcluster)  [unwired: 5 in, 1 out]
        n100 = property on="Select device" class="CmbBox"("Strings[]"=w209) -> ()  [unwired: 2 in, 2 out]
        n101 = call <vilib>:"Add State(s) to Queue__jki_lib_state_machine.vi"("State(s) in (\"\")"=w215) -> ("States Out"=w214:string)  [unwired: 14 in]
      }
      frame "UI: Get Device Name" {
        # "Initialize the User Interface, here.\n(this is called automatically, by the Macro: Init)"
        n102 = First Call?() -> (First Call?: T/F=w220:bool)
        n103 = case shown="True" w220 {
          tunnel: w219 -> [w224 w226]
          tunnel: [w224 w225] -> w218
          frame False {
          }
          frame True {
            n104 = disable-structure "Get Device name from control for vi mode\nand command line arg for exe" shown="RUN_TIME_ENGINE==True" {
              disable-tunnel: w226 -> [w227 w229]
              disable-tunnel: [w227 w228] -> w225
              frame condition #0 (active) {
              }
              frame condition #1 {
                n105 = control-ref of="This Application"() -> (w237:refnum<vi>)
                n106 = property class="App"(reference=w237) -> ("App.Args"=w236:string[])  [unwired: 1 in, 2 out]
                n107 = Index Array(array=w236, index #1=1 ("index")) -> (element #1=w230:string)  [unwired: 2 in, 2 out]
                n108 = Empty String/Path?(string/path=w230) -> (empty?=w234:bool)
                n109 = control-ref of="This VI"() -> (w233:refnum<vi>)
                n110 = case shown="False" w234 {
                  tunnel: w230 -> [w238 _]
                  frame False {
                    n111 = local write "GUIdevice 1"(w238) -> ()
                  }
                  frame True {
                  }
                }
                n112 = Concatenate Strings(w230, "_GUI ") -> (w232:string)
                n113 = property class="VI"(reference=w233, error in=w229, "Front Panel.Title"=w232) -> (error out=w228:errorcluster)  [unwired: 1 out]
              }
            }
          }
        }
        n114 = call <vilib>:"Add State(s) to Queue__jki_lib_state_machine.vi"("State(s) in (\"\")"=w223) -> ("States Out"=w222:string)  [unwired: 14 in]
      }
      frame "UI: Start SuperGUI" {
        # "create stop queue for supergui and its clones"
        # "x100 abort will be dependent on caller VI\nx80 abort will be independent of caller vi, this will abort vi when labview is closed."
        # "Start SuperGUI asynchronous way"
        n115 = vi-ref "GUI_Master_subvi_reentrant_queues.vi"() -> (w241:refnum<vi>)
        n116 = property class="VI"(reference=w241) -> ("Path"=w240:path)  [unwired: 1 in, 2 out]
        n117 = Create User Event(user event datatype=T23 {"EventEnum"=enum."new data", "Device name"="Device name"} ("New Event"), error in=w243) -> (user event=w244:refnum<user-event>, error out=w250:errorcluster)
        "tcp data event" <- w244
        n118 = control-ref of="This Application"() -> (w247:refnum<vi>)
        n119 = control-ref of="This VI"() -> (w246:refnum<vi>)
        n120 = Open VI Reference(type specifier VI Refnum (for type only)=refnum<vi> refnum, vi path=w240, options=256) -> (vi reference=w256:refnum<vi>, error out=w255:errorcluster)  [unwired: 3 in]
        n121 = register-events(w244) -> ()  [unwired: 2 in, 2 out]
        n122 = call "supergui create stop queue.vi"() -> ("STOP Queue out"=w252:refnum<queue>)  [unwired: 11 in]
        n123 = Current VI's Menubar() -> (w245:refnum<k9>)
        n124 = call-by-ref "Start Asynchronous Call"(reference=w256, error in=w255, "STOP Queue in"=w252, "This Application"=w247, 8:"error in (no error)"=w250, "tcp data event"=w244, "Caller menu reference"=w245, "Caller VI ref"=w246) -> (reference out=w239:refnum<vi>, error out=w242:errorcluster)  [unwired: 5 in, 1 out]
        n125 = Bundle By Name(cluster=w249, "SuperGUI.SuperGUI ref"=w239, "SuperGUI.STOP queue"=w252) -> (w248:T25)
        n126 = call <vilib>:"Add State(s) to Queue__jki_lib_state_machine.vi"("State(s) in (\"\")"=w258) -> ("States Out"=w257:string)  [unwired: 14 in]
      }
      frame "UI: Stop SuperGUI" {
        # "Stop Supergui Clone and wait until it exit properly"
        n127 = Unbundle By Name(w261) -> ("SuperGUI.SuperGUI ref"=w263:refnum<vi>, "SuperGUI.STOP queue"=w262:refnum<queue>)
        n128 = Release Queue(queue=w262, error in (no error)=w260) -> (error out=w264:errorcluster)  [unwired: 1 in, 2 out]
        n129 = call-by-ref "Wait On Asynchronous Call"(reference=w263, error in=w264) -> ("error out"=w259:errorcluster)  [unwired: 11 in, 2 out]
        n130 = call <vilib>:"Add State(s) to Queue__jki_lib_state_machine.vi"("State(s) in (\"\")"=w266) -> ("States Out"=w265:string)  [unwired: 14 in]
      }
      frame "UI: Cursor Set" {
        # "Argument"
        # "Set and Unset Cursor Busy.\n(Usage: \"UI: Cursor Set >> Busy|Idle\")"
        n131 = case shown="\"Idle\", Default" w267 {
          tunnel: w269 -> [w274 w276]
          tunnel: [w273 w275] -> w268
          frame "Idle", Default {
            n132 = call <vilib>:"Unset Busy.vi"("error in (no error)"=w274) -> ("error out"=w273:errorcluster)  [unwired: 10 in]
          }
          frame "Busy" {
            n133 = call <vilib>:"Set Busy.vi"("error in (no error)"=w276) -> ("error out"=w275:errorcluster)  [unwired: 9 in, 1 out]
          }
        }
        n134 = call <vilib>:"Add State(s) to Queue__jki_lib_state_machine.vi"("State(s) in (\"\")"=w272) -> ("States Out"=w271:string)  [unwired: 14 in]
      }
      frame "UI: Front Panel State" {
        # "Argument"
        # "Set Front Panel Open or Closed\n(Usage: \"UI: Front Panel State >> Open|Close\")"
        n135 = Unbundle By Name(w279) -> ("Core.Current VI Reference"=w278:refnum<vi>)
        n136 = case shown="\"Open\", Default" w277 {
          tunnel: w281 -> [w287 w300]
          tunnel: [w289 w301] -> w280
          tunnel: w278 -> [w288 w298]
          frame "Open", Default {
            n137 = property class="VI"(reference=w288, error in=w287) -> (reference out=w285:refnum<vi>, error out=w286:errorcluster, "Front Panel.Open"=w284:bool)
            n138 = case shown="False" w284 {
              tunnel: [w292 w295] -> w289
              tunnel: w286 -> [w291 w295]
              tunnel: w285 -> [w290 _]
              frame False {
                n139 = invoke class="VI" method="FP.Open"(reference=w290, error in=w291, "Activate"=TRUE, "State"=T24."Standard") -> (error out=w292:errorcluster)  [unwired: 1 in, 4 out]
              }
              frame True {
              }
            }
          }
          frame "Close" {
            n140 = property class="VI"(reference=w298, error in=w300) -> (reference out=w297:refnum<vi>, error out=w299:errorcluster, "Front Panel.Open"=w296:bool)
            n141 = case shown="True" w296 {
              tunnel: [w302 w305] -> w301
              tunnel: w299 -> [w302 w304]
              tunnel: w297 -> [_ w303]
              frame False {
              }
              frame True {
                n142 = invoke class="VI" method="FP.Close"(reference=w303, error in=w304) -> (error out=w305:errorcluster)  [unwired: 1 in, 2 out]
              }
            }
          }
        }
        n143 = call <vilib>:"Add State(s) to Queue__jki_lib_state_machine.vi"("State(s) in (\"\")"=w283) -> ("States Out"=w282:string)  [unwired: 14 in]
      }
      frame "---------- Macro ----------" {
        # "Do not put any code in this frame.\n(It is a separator no-op. You can make a copy of this frame to create a new Macro frame)"
        n144 = call <vilib>:"Add State(s) to Queue__jki_lib_state_machine.vi"("State(s) in (\"\")"=w309) -> ("States Out"=w308:string)  [unwired: 14 in]
      }
      frame "Macro: Initialize" {
        # "Initialization Macro\n(This is called once, when the VI starts)"
        n145 = call <vilib>:"Add State(s) to Queue__jki_lib_state_machine.vi"("State(s) in Front (\"\")"="Data: Initialize\nInitialize Core Data\nUI: Initialize\nUI: Get Device Name\nUI: Start SuperGUI\nUI: Front Panel State >> Open", "State(s) in (\"\")"=w314) -> ("States Out"=w313:string)  [unwired: 13 in]
      }
      frame "Macro: Exit" {
        # "Exit Macro\n(This is called once, when the VI exits)"
        n146 = Unbundle By Name(w321) -> ("Core.Close Panel on Exit?"=w320:bool)
        n147 = Select(t="UI: Front Panel State >> Close", s=w320, f="") -> (s? t:f=w317:string)
        n148 = call <vilib>:"Add State(s) to Queue__jki_lib_state_machine.vi"("State(s) in (\"\")"=w317, "State(s) at Back (\"\")"="Data: Cleanup\nExit") -> ("States Out"=w315:string)  [unwired: 13 in]
        n149 = call <vilib>:"Add State(s) to Queue__jki_lib_state_machine.vi"("State(s) in Front (\"\")"=w315, "State(s) in (\"\")"=w324) -> ("States Out"=w323:string)  [unwired: 13 in]
      }
      frame "---------- New Category ----------" {
        # "Template Separator\n(You can make a copy of, or modify, this frame)"
        n150 = call <vilib>:"Add State(s) to Queue__jki_lib_state_machine.vi"("State(s) in (\"\")"=w328) -> ("States Out"=w327:string)  [unwired: 14 in]
      }
      frame "New Category: 1" {
        # "Your code here.\n(You can make a copy of, or modify, this frame)"
        n151 = call <vilib>:"Add State(s) to Queue__jki_lib_state_machine.vi"("State(s) in (\"\")"=w332) -> ("States Out"=w331:string)  [unwired: 14 in]
      }
      frame "New Category: 2" {
        # "Your code here.\n(You can make a copy of, or modify, this frame)"
        n152 = call <vilib>:"Add State(s) to Queue__jki_lib_state_machine.vi"("State(s) in (\"\")"=w336) -> ("States Out"=w335:string)  [unwired: 14 in]
      }
    }
    n153 = for {
      tunnel: w60 -> [w87]
      tunnel: w59 -> [w91]
      tunnel: w57 -> [w88] mode=indexing
      tunnel: w56 -> [w84]
      (unwired) u32 16774656 ("Color")
      n154 = call-poly <userlib>:"Filter 1D Array__ogtk.vi"("items to filter"=w88, "array"=w91) -> ("filtered item indices"=w92:i32[])  [unwired: 4 in, 1 out]
      n155 = Index Array(array=w92) -> (element=w86:i32)  [unwired: 1 in]
      n156 = Index Array(array=w84, index=w86) -> (element=w85:T10)
      n157 = Unbundle By Name(w85) -> ("TargetSize.X::7"=w83:refnum<vi>, "TargetSize.Y::7"=w82:refnum<vi>)
      n158 = Index Array(array=w87, index=w86) -> (element=w90:T16)
      n159 = property class="DigNum (strict)"(reference=w83) -> ("Value"=w81:dbl)  [unwired: 1 in, 2 out]
      n160 = property class="DigNum (strict)"(reference=w82) -> ("Value"=w80:dbl)  [unwired: 1 in, 2 out]
      n161 = Unbundle By Name(w90) -> ("Target.X::7"=w94:refnum<vi>, "Target.Y::7"=w93:refnum<vi>)
      n162 = property class="DigNum (strict)"(reference=w94) -> ("Value"=w76:dbl)  [unwired: 1 in, 2 out]
      n163 = property class="DigNum (strict)"(reference=w93) -> ("Value"=w75:dbl)  [unwired: 1 in, 2 out]
      n164 = Bundle("Value"=w76, "Value"=w75) -> (w74:cluster{"Value":dbl, "Value":dbl})  [unwired: 1 in]
      n165 = Bundle("Value"=w81, "Value"=w80) -> (w73:cluster{"Value":dbl, "Value":dbl})  [unwired: 1 in]
      n166 = Bundle By Name(cluster=T20 {"Draw"=TRUE, "Target"={"x"=20.0, "y"=20.0}, "Size"={"x"=20.0, "y"=20.0}, "Angle"=1250067.0, "Color"=1250067} ("Crosshair"), "Draw"=TRUE, "Target"=w74, "Size"=w73, "Angle"=0.0, "Color"="Color Box") -> (w78:T20)
      n167 = call "draw crosshair imaq.vi"("Crosshair"=w78, "Bounding Rectangle"=T21 {"Left"=0, "Top"=0, "Right"=0, "Bottom"=0}, "image in"=w88) -> ("error out"=→"error out":errorcluster)  [unwired: 7 in, 1 out]
    }
  }
